vi "Pop.vi"(11 "POTTypedCircularBuffer in":refnum<class "POTTypedCircularBuffer.lvclass">) -> (1 "invalid?":bool, 2 "element":T1, 3 "POTTypedCircularBuffer out":refnum<class "POTTypedCircularBuffer.lvclass">)   [LabVIEW 2024, in "POTTypedCircularBuffer.lvclass"]
uses:
  POTTypedCircularBuffer.lvclass
  Type.ctl
  POTTypedCircularBuffer.lvclass/POTTypedCircularBuffer.ctl
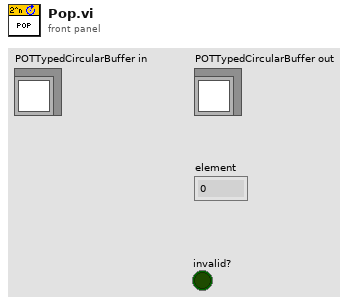
[diagram p1: front panel]
types:
  T1 = typedef "POTTypedCircularBuffer.lvclass/Type.ctl" = i32
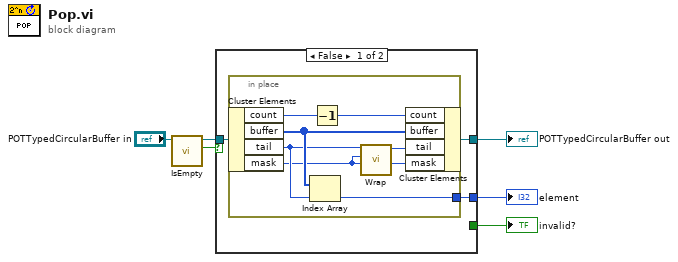
[diagram p0: block diagram]
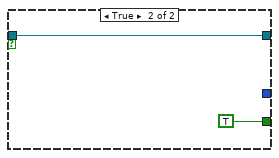
[diagram p2: hidden frame]
diagram:
  n1 = call "IsEmpty.vi"("POTTypedCircularBuffer in"="POTTypedCircularBuffer in") -> ("Empty?"=w3:bool, "POTTypedCircularBuffer out"=w1:refnum<class "POTTypedCircularBuffer.lvclass">)  [unwired: 9 in]
  n2 = case shown="False" w3 {
    tunnel: w1 -> [w9 w18]
    tunnel: [w8 _] -> w5
    tunnel: [w7 w18] -> w6
    tunnel: [_ TRUE] -> w4
    frame False {
      n3 = in-place {
        in-place-border: [w16] -> w8
        n4 = in-place-cluster #1(w9) -> ("count"=w14:i32, "buffer"=w15:T1[], "tail"=w12:i32, "mask"=w11:i32)
        n5 = Index Array(array=w15, index=w12) -> (element=w16:T1)
        n6 = Decrement(x=w14) -> (x-1=w13:i32)
        n7 = call "Wrap.vi"("mask"=w11, "index"=w12) -> ("wrapped"=w10:i32)  [unwired: 9 in]
        n8 = in-place-cluster #1("count"=w13, "buffer"=w15, "tail"=w10, "mask"=w11) -> (w7:refnum<class "POTTypedCircularBuffer.lvclass">)
      }
    }
    frame True {
    }
  }
  "POTTypedCircularBuffer out" <- w6
  "element" <- w5
  "invalid?" <- w4
